vi "S4GUI.vi"(7 "Tab ObsEng":enum32{"Obs", "CCD modes", "Eng"}(tab)) -> ()   [LabVIEW 2018] (continued)
        n3639 = call-dynamic "Read Channel.vi"("error in (no error)"=w8486, "Acquisition in"=w8487) -> ("error out"=w8475:errorcluster, "Channel.lvclass"=w8476:refnum<class "Channel.lvclass">, "Acquisition out"=w8477:refnum<class "Acquisition.lvclass">)  [unwired: 7 in]
        n3640 = call-dynamic "Read Interface.vi"("error in (no error)"=w8475, "Channel in"=w8476) -> ("error out"=w8481:errorcluster, "Interface.lvclass"=w8482:refnum<class "Interface.lvclass">, "Channel out"=w8480:refnum<class "Channel.lvclass">)  [unwired: 7 in]
        n3641 = call "Write Exposure Time.vi"("error in (no error)"=w8481, "Exposure Time"=w8472, "Interface in"=w8482) -> ("error out"=w8473:errorcluster, "Interface out"=w8474:refnum<class "Interface.lvclass">)  [unwired: 7 in]
        n3642 = call-dynamic "Write Interface.vi"("error in (no error)"=w8473, "Interface.lvclass"=w8474, "Channel in"=w8480) -> ("error out"=w8479:errorcluster, "Channel out"=w8478:refnum<class "Channel.lvclass">)  [unwired: 7 in]
        n3643 = call-dynamic "Write Channel.vi"("error in (no error)"=w8479, "Channel.lvclass"=w8478, "Acquisition in"=w8477) -> ("error out"=w8483:errorcluster, "Acquisition out"=w8485:refnum<class "Acquisition.lvclass">)  [unwired: 7 in]
        n3644 = call-dynamic "Write AcquisitionD.vi"("error in (no error)"=w8483, "Acquisition.lvclass"=w8485, "S4ACS_GUI in"=w8484) -> ("error out"=w8469:errorcluster, "S4ACS_GUI out"=w8468:refnum<class "S4GUI.lvclass">)  [unwired: 7 in]
      }
      event "Stop ch1": Value Change {
        n3645 = event-data() -> ()  [unwired: 1 in, 6 out]
        n3646 = disable-structure shown="Enabled" {
          disable-tunnel: w8491 -> [w8524 w8552]
          disable-tunnel: w8490 -> [w8522 w8546]
          disable-tunnel: [w8504 w8545] -> w8489
          disable-tunnel: [w8492 w8552] -> w8488
          frame Disabled {
            # "Para movimento \nda lamina retardadora"
            # "Restaura a última sequência de lâminas"
            n3647 = call-dynamic "Read AcquisitionA.vi"("error in (no error)"=w8522, "S4ACS_GUI in"=w8524) -> ("error out"=w8526:errorcluster, "Acquisition.lvclass"=w8525:refnum<class "Acquisition.lvclass">, "S4ACS_GUI out"=w8523:refnum<class "S4GUI.lvclass">)  [unwired: 7 in]
            n3648 = disable-structure shown="Enabled" {
              disable-tunnel: w8526 -> [w8531 w8542]
              disable-tunnel: w8525 -> [w8530 w8543]
              disable-tunnel: [w8528 w8543] -> w8520
              disable-tunnel: [w8527 w8542] -> w8519
              frame Disabled {
                # "Só precisa enviar comando STOP quando\no controle dos ciclos for feito pelo ACS."
                n3649 = call-dynamic "Read Channel.vi"("error in (no error)"=w8531, "Acquisition in"=w8530) -> ("error out"=w8533:errorcluster, "Channel.lvclass"=w8532:refnum<class "Channel.lvclass">, "Acquisition out"=w8539:refnum<class "Acquisition.lvclass">)  [unwired: 7 in]
                n3650 = call-dynamic "Read State Machine.vi"("error in (no error)"=w8533, "Device in"=w8532) -> ("error out"=w8535:errorcluster, "State Machine.lvclass"=w8534:refnum<class "State Machine.lvclass">, "Device out"=w8537:refnum<class "Channel.lvclass">)  [unwired: 7 in]
                n3651 = call "Next State.vi"("error in (no error)"=w8535, "New_State"=u32 70, "State Machine in"=w8534) -> ("error out"=w8538:errorcluster, "State Machine out"=w8536:refnum<class "State Machine.lvclass">)  [unwired: 7 in]
                n3652 = call-dynamic "Write State Machine.vi"("error in (no error)"=w8538, "State Machine.lvclass"=w8536, "Device in"=w8537) -> ("error out"=w8540:errorcluster, "Device out"=w8541:refnum<class "Channel.lvclass">)  [unwired: 7 in]
                n3653 = call-dynamic "Write Channel.vi"("error in (no error)"=w8540, "Channel.lvclass"=w8541, "Acquisition in"=w8539) -> ("error out"=w8527:errorcluster, "Acquisition out"=w8528:refnum<class "Acquisition.lvclass">)  [unwired: 7 in]
              }
              frame Enabled {
                # "Não precisa enviar comando STOP para o ACS\nenquanto o controle dos ciclos for feito pela GUI."
              }
            }
            n3654 = call-dynamic "Write Acq_state.vi"("error in (no error)"=w8519, "Acq_state"=u32 0, "Acquisition in"=w8520) -> ("error out"=w8518:errorcluster, "Acquisition out"=w8517:refnum<class "Acquisition.lvclass">)  [unwired: 7 in]
            n3655 = call-dynamic "Write AcquisitionA.vi"("error in (no error)"=w8518, "Acquisition.lvclass"=w8517, "S4ACS_GUI in"=w8523) -> ("error out"=w8505:errorcluster, "S4ACS_GUI out"=w8503:refnum<class "S4GUI.lvclass">)  [unwired: 7 in]
            n3656 = call "Read Instrument.lvclass.vi"("error in (no error)"=w8505, "S4ACS_GUI in"=w8503) -> ("error out"=w8512:errorcluster, "Instrument.lvclass"=w8515:refnum<class "Instrument.lvclass">, "S4ACS_GUI out"=w8516:refnum<class "S4GUI.lvclass">)  [unwired: 7 in]
            n3657 = call "Read WPROT.vi"("error in (no error)"=w8512, "Instrument in"=w8515) -> ("error out"=w8511:errorcluster, "Opt_Selector.lvclass"=w8513:refnum<class "Opt_Selector.lvclass">, "Instrument out"=w8514:refnum<class "Instrument.lvclass">)  [unwired: 7 in]
            n3658 = call-dynamic "Read sequencia_ant.vi"("error in (no error)"=w8511, "Opt_Selector in"=w8513) -> ("error out"=w8507:errorcluster, "sequencia_ant"=w8506:u16, "Opt_Selector out"=w8508:refnum<class "Opt_Selector.lvclass">)  [unwired: 7 in]
            n3659 = call-dynamic "Write sequencia.vi"("error in (no error)"=w8507, "sequencia"=w8506, "Opt_Selector in"=w8508) -> ("error out"=w8494:errorcluster, "Opt_Selector out"=w8497:refnum<class "Opt_Selector.lvclass">)  [unwired: 7 in]
            n3660 = call-dynamic "Read State Machine.vi"("error in (no error)"=w8494, "Device in"=w8497) -> ("error out"=w8499:errorcluster, "State Machine.lvclass"=w8502:refnum<class "State Machine.lvclass">, "Device out"=w8496:refnum<class "Opt_Selector.lvclass">)  [unwired: 7 in]
            n3661 = call "Next State.vi"("error in (no error)"=w8499, "New_State"=10, "State Machine in"=w8502) -> ("error out"=w8498:errorcluster, "State Machine out"=w8501:refnum<class "State Machine.lvclass">)  [unwired: 7 in]
            n3662 = call-dynamic "Write State Machine.vi"("error in (no error)"=w8498, "State Machine.lvclass"=w8501, "Device in"=w8496) -> ("error out"=w8493:errorcluster, "Device out"=w8495:refnum<class "Opt_Selector.lvclass">)  [unwired: 7 in]
            n3663 = call "Write WPROT.vi"("error in (no error)"=w8493, "Opt_Selector.lvclass"=w8495, "Instrument in"=w8514) -> ("error out"=w8510:errorcluster, "Instrument out"=w8509:refnum<class "Instrument.lvclass">)  [unwired: 7 in]
            n3664 = call "Write Instrument.lvclass.vi"("error in (no error)"=w8510, "Instrument.lvclass"=w8509, "S4ACS_GUI in"=w8516) -> ("error out"=w8504:errorcluster, "S4ACS_GUI out"=w8492:refnum<class "S4GUI.lvclass">)  [unwired: 7 in]
          }
          frame Enabled {
            w8548 = FALSE ("Wait Until Done")
            n3665 = call <vilib>:"Application Directory.vi"() -> ("Application Directory"=w8544:path)
            n3666 = Build Path(base path=w8544, name or relative path="MsgStop1.vi") -> (appended path=w8551:path)
            n3667 = Open VI Reference(vi path=w8551, error in (no error)=w8546) -> (vi reference=w8550:refnum<vi>, error out=w8549:errorcluster)  [unwired: 4 in]
            n3668 = invoke class="VI" method="Run VI"(reference=w8550, error in=w8549, "Wait until done"=w8548, "Auto Dispose Ref"=w8548) -> (error out=w8545:errorcluster)  [unwired: 1 in, 4 out]
          }
        }
      }
      event "Stop ch2": Value Change {
        n3669 = event-data() -> ()  [unwired: 1 in, 6 out]
        n3670 = disable-structure shown="Enabled" {
          disable-tunnel: w8556 -> [w8589 w8610]
          disable-tunnel: w8555 -> [w8587 w8612]
          disable-tunnel: [w8569 w8611] -> w8554
          disable-tunnel: [w8557 w8610] -> w8553
          frame Disabled {
            # "Para movimento \nda lamina retardadora"
            # "Restaura a última sequência de lâminas"
            n3671 = call "Read AcquisitionB.vi"("error in (no error)"=w8587, "S4ACS_GUI in"=w8589) -> ("error out"=w8591:errorcluster, "Acquisition.lvclass"=w8590:refnum<class "Acquisition.lvclass">, "S4ACS_GUI out"=w8588:refnum<class "S4GUI.lvclass">)  [unwired: 7 in]
            n3672 = disable-structure shown="Enabled" {
              disable-tunnel: w8591 -> [w8596 w8607]
              disable-tunnel: w8590 -> [w8595 w8608]
              disable-tunnel: [w8593 w8608] -> w8585
              disable-tunnel: [w8592 w8607] -> w8584
              frame Disabled {
                # "Só precisa enviar comando STOP quando\no controle dos ciclos for feito pelo ACS."
                n3673 = call-dynamic "Read Channel.vi"("error in (no error)"=w8596, "Acquisition in"=w8595) -> ("error out"=w8598:errorcluster, "Channel.lvclass"=w8597:refnum<class "Channel.lvclass">, "Acquisition out"=w8604:refnum<class "Acquisition.lvclass">)  [unwired: 7 in]
                n3674 = call-dynamic "Read State Machine.vi"("error in (no error)"=w8598, "Device in"=w8597) -> ("error out"=w8600:errorcluster, "State Machine.lvclass"=w8599:refnum<class "State Machine.lvclass">, "Device out"=w8602:refnum<class "Channel.lvclass">)  [unwired: 7 in]
                n3675 = call "Next State.vi"("error in (no error)"=w8600, "New_State"=u32 70, "State Machine in"=w8599) -> ("error out"=w8603:errorcluster, "State Machine out"=w8601:refnum<class "State Machine.lvclass">)  [unwired: 7 in]
                n3676 = call-dynamic "Write State Machine.vi"("error in (no error)"=w8603, "State Machine.lvclass"=w8601, "Device in"=w8602) -> ("error out"=w8605:errorcluster, "Device out"=w8606:refnum<class "Channel.lvclass">)  [unwired: 7 in]
                n3677 = call-dynamic "Write Channel.vi"("error in (no error)"=w8605, "Channel.lvclass"=w8606, "Acquisition in"=w8604) -> ("error out"=w8592:errorcluster, "Acquisition out"=w8593:refnum<class "Acquisition.lvclass">)  [unwired: 7 in]
              }
              frame Enabled {
                # "Não precisa enviar comando STOP para o ACS\nenquanto o controle dos ciclos for feito pela GUI."
              }
            }
            n3678 = call-dynamic "Write Acq_state.vi"("error in (no error)"=w8584, "Acq_state"=u32 0, "Acquisition in"=w8585) -> ("error out"=w8583:errorcluster, "Acquisition out"=w8582:refnum<class "Acquisition.lvclass">)  [unwired: 7 in]
            n3679 = call "Write AcquisitionB.vi"("error in (no error)"=w8583, "Acquisition.lvclass"=w8582, "S4ACS_GUI in"=w8588) -> ("error out"=w8570:errorcluster, "S4ACS_GUI out"=w8568:refnum<class "S4GUI.lvclass">)  [unwired: 7 in]
            n3680 = call "Read Instrument.lvclass.vi"("error in (no error)"=w8570, "S4ACS_GUI in"=w8568) -> ("error out"=w8577:errorcluster, "Instrument.lvclass"=w8580:refnum<class "Instrument.lvclass">, "S4ACS_GUI out"=w8581:refnum<class "S4GUI.lvclass">)  [unwired: 7 in]
            n3681 = call "Read WPROT.vi"("error in (no error)"=w8577, "Instrument in"=w8580) -> ("error out"=w8576:errorcluster, "Opt_Selector.lvclass"=w8578:refnum<class "Opt_Selector.lvclass">, "Instrument out"=w8579:refnum<class "Instrument.lvclass">)  [unwired: 7 in]
            n3682 = call-dynamic "Read sequencia_ant.vi"("error in (no error)"=w8576, "Opt_Selector in"=w8578) -> ("error out"=w8572:errorcluster, "sequencia_ant"=w8571:u16, "Opt_Selector out"=w8573:refnum<class "Opt_Selector.lvclass">)  [unwired: 7 in]
            n3683 = call-dynamic "Write sequencia.vi"("error in (no error)"=w8572, "sequencia"=w8571, "Opt_Selector in"=w8573) -> ("error out"=w8559:errorcluster, "Opt_Selector out"=w8562:refnum<class "Opt_Selector.lvclass">)  [unwired: 7 in]
            n3684 = call-dynamic "Read State Machine.vi"("error in (no error)"=w8559, "Device in"=w8562) -> ("error out"=w8564:errorcluster, "State Machine.lvclass"=w8567:refnum<class "State Machine.lvclass">, "Device out"=w8561:refnum<class "Opt_Selector.lvclass">)  [unwired: 7 in]
            n3685 = call "Next State.vi"("error in (no error)"=w8564, "New_State"=10, "State Machine in"=w8567) -> ("error out"=w8563:errorcluster, "State Machine out"=w8566:refnum<class "State Machine.lvclass">)  [unwired: 7 in]
            n3686 = call-dynamic "Write State Machine.vi"("error in (no error)"=w8563, "State Machine.lvclass"=w8566, "Device in"=w8561) -> ("error out"=w8558:errorcluster, "Device out"=w8560:refnum<class "Opt_Selector.lvclass">)  [unwired: 7 in]
            n3687 = call "Write WPROT.vi"("error in (no error)"=w8558, "Opt_Selector.lvclass"=w8560, "Instrument in"=w8579) -> ("error out"=w8575:errorcluster, "Instrument out"=w8574:refnum<class "Instrument.lvclass">)  [unwired: 7 in]
            n3688 = call "Write Instrument.lvclass.vi"("error in (no error)"=w8575, "Instrument.lvclass"=w8574, "S4ACS_GUI in"=w8581) -> ("error out"=w8569:errorcluster, "S4ACS_GUI out"=w8557:refnum<class "S4GUI.lvclass">)  [unwired: 7 in]
          }
          frame Enabled {
            w8614 = FALSE ("Wait Until Done")
            n3689 = call <vilib>:"Application Directory.vi"() -> ("Application Directory"=w8609:path)
            n3690 = Build Path(base path=w8609, name or relative path="MsgStop2.vi") -> (appended path=w8617:path)
            n3691 = Open VI Reference(vi path=w8617, error in (no error)=w8612) -> (vi reference=w8616:refnum<vi>, error out=w8615:errorcluster)  [unwired: 4 in]
            n3692 = invoke class="VI" method="Run VI"(reference=w8616, error in=w8615, "Wait until done"=w8614, "Auto Dispose Ref"=w8614) -> (error out=w8611:errorcluster)  [unwired: 1 in, 4 out]
          }
        }
      }
      event "Stop ch3": Value Change {
        n3693 = event-data() -> ()  [unwired: 1 in, 6 out]
        n3694 = disable-structure shown="Enabled" {
          disable-tunnel: w8621 -> [w8654 w8675]
          disable-tunnel: w8620 -> [w8652 w8677]
          disable-tunnel: [w8634 w8676] -> w8619
          disable-tunnel: [w8622 w8675] -> w8618
          frame Disabled {
            # "Para movimento \nda lamina retardadora"
            # "Restaura a última sequência de lâminas"
            n3695 = call-dynamic "Read AcquisitionC.vi"("error in (no error)"=w8652, "S4ACS_GUI in"=w8654) -> ("error out"=w8656:errorcluster, "Acquisition.lvclass"=w8655:refnum<class "Acquisition.lvclass">, "S4ACS_GUI out"=w8653:refnum<class "S4GUI.lvclass">)  [unwired: 7 in]
            n3696 = disable-structure shown="Enabled" {
              disable-tunnel: w8656 -> [w8661 w8672]
              disable-tunnel: w8655 -> [w8660 w8673]
              disable-tunnel: [w8658 w8673] -> w8650
              disable-tunnel: [w8657 w8672] -> w8649
              frame Disabled {
                # "Só precisa enviar comando STOP quando\no controle dos ciclos for feito pelo ACS."
                n3697 = call-dynamic "Read Channel.vi"("error in (no error)"=w8661, "Acquisition in"=w8660) -> ("error out"=w8663:errorcluster, "Channel.lvclass"=w8662:refnum<class "Channel.lvclass">, "Acquisition out"=w8669:refnum<class "Acquisition.lvclass">)  [unwired: 7 in]
                n3698 = call-dynamic "Read State Machine.vi"("error in (no error)"=w8663, "Device in"=w8662) -> ("error out"=w8665:errorcluster, "State Machine.lvclass"=w8664:refnum<class "State Machine.lvclass">, "Device out"=w8667:refnum<class "Channel.lvclass">)  [unwired: 7 in]
                n3699 = call "Next State.vi"("error in (no error)"=w8665, "New_State"=u32 70, "State Machine in"=w8664) -> ("error out"=w8668:errorcluster, "State Machine out"=w8666:refnum<class "State Machine.lvclass">)  [unwired: 7 in]
                n3700 = call-dynamic "Write State Machine.vi"("error in (no error)"=w8668, "State Machine.lvclass"=w8666, "Device in"=w8667) -> ("error out"=w8670:errorcluster, "Device out"=w8671:refnum<class "Channel.lvclass">)  [unwired: 7 in]
                n3701 = call-dynamic "Write Channel.vi"("error in (no error)"=w8670, "Channel.lvclass"=w8671, "Acquisition in"=w8669) -> ("error out"=w8657:errorcluster, "Acquisition out"=w8658:refnum<class "Acquisition.lvclass">)  [unwired: 7 in]
              }
              frame Enabled {
                # "Não precisa enviar comando STOP para o ACS\nenquanto o controle dos ciclos for feito pela GUI."
              }
            }
            n3702 = call-dynamic "Write Acq_state.vi"("error in (no error)"=w8649, "Acq_state"=u32 0, "Acquisition in"=w8650) -> ("error out"=w8648:errorcluster, "Acquisition out"=w8647:refnum<class "Acquisition.lvclass">)  [unwired: 7 in]
            n3703 = call-dynamic "Write AcquisitionC.vi"("error in (no error)"=w8648, "Acquisition.lvclass"=w8647, "S4ACS_GUI in"=w8653) -> ("error out"=w8635:errorcluster, "S4ACS_GUI out"=w8633:refnum<class "S4GUI.lvclass">)  [unwired: 7 in]
            n3704 = call "Read Instrument.lvclass.vi"("error in (no error)"=w8635, "S4ACS_GUI in"=w8633) -> ("error out"=w8642:errorcluster, "Instrument.lvclass"=w8645:refnum<class "Instrument.lvclass">, "S4ACS_GUI out"=w8646:refnum<class "S4GUI.lvclass">)  [unwired: 7 in]
            n3705 = call "Read WPROT.vi"("error in (no error)"=w8642, "Instrument in"=w8645) -> ("error out"=w8641:errorcluster, "Opt_Selector.lvclass"=w8643:refnum<class "Opt_Selector.lvclass">, "Instrument out"=w8644:refnum<class "Instrument.lvclass">)  [unwired: 7 in]
            n3706 = call-dynamic "Read sequencia_ant.vi"("error in (no error)"=w8641, "Opt_Selector in"=w8643) -> ("error out"=w8637:errorcluster, "sequencia_ant"=w8636:u16, "Opt_Selector out"=w8638:refnum<class "Opt_Selector.lvclass">)  [unwired: 7 in]
            n3707 = call-dynamic "Write sequencia.vi"("error in (no error)"=w8637, "sequencia"=w8636, "Opt_Selector in"=w8638) -> ("error out"=w8624:errorcluster, "Opt_Selector out"=w8627:refnum<class "Opt_Selector.lvclass">)  [unwired: 7 in]
            n3708 = call-dynamic "Read State Machine.vi"("error in (no error)"=w8624, "Device in"=w8627) -> ("error out"=w8629:errorcluster, "State Machine.lvclass"=w8632:refnum<class "State Machine.lvclass">, "Device out"=w8626:refnum<class "Opt_Selector.lvclass">)  [unwired: 7 in]
            n3709 = call "Next State.vi"("error in (no error)"=w8629, "New_State"=10, "State Machine in"=w8632) -> ("error out"=w8628:errorcluster, "State Machine out"=w8631:refnum<class "State Machine.lvclass">)  [unwired: 7 in]
            n3710 = call-dynamic "Write State Machine.vi"("error in (no error)"=w8628, "State Machine.lvclass"=w8631, "Device in"=w8626) -> ("error out"=w8623:errorcluster, "Device out"=w8625:refnum<class "Opt_Selector.lvclass">)  [unwired: 7 in]
            n3711 = call "Write WPROT.vi"("error in (no error)"=w8623, "Opt_Selector.lvclass"=w8625, "Instrument in"=w8644) -> ("error out"=w8640:errorcluster, "Instrument out"=w8639:refnum<class "Instrument.lvclass">)  [unwired: 7 in]
            n3712 = call "Write Instrument.lvclass.vi"("error in (no error)"=w8640, "Instrument.lvclass"=w8639, "S4ACS_GUI in"=w8646) -> ("error out"=w8634:errorcluster, "S4ACS_GUI out"=w8622:refnum<class "S4GUI.lvclass">)  [unwired: 7 in]
          }
          frame Enabled {
            w8679 = FALSE ("Wait Until Done")
            n3713 = call <vilib>:"Application Directory.vi"() -> ("Application Directory"=w8674:path)
            n3714 = Build Path(base path=w8674, name or relative path="MsgStop3.vi") -> (appended path=w8682:path)
            n3715 = Open VI Reference(vi path=w8682, error in (no error)=w8677) -> (vi reference=w8681:refnum<vi>, error out=w8680:errorcluster)  [unwired: 4 in]
            n3716 = invoke class="VI" method="Run VI"(reference=w8681, error in=w8680, "Wait until done"=w8679, "Auto Dispose Ref"=w8679) -> (error out=w8676:errorcluster)  [unwired: 1 in, 4 out]
          }
        }
      }
      event "Stop ch4": Value Change {
        n3717 = event-data() -> ()  [unwired: 1 in, 6 out]
        n3718 = disable-structure shown="Enabled" {
          disable-tunnel: w8686 -> [w8719 w8740]
          disable-tunnel: w8685 -> [w8717 w8742]
          disable-tunnel: [w8699 w8741] -> w8684
          disable-tunnel: [w8687 w8740] -> w8683
          frame Disabled {
            # "Para movimento \nda lamina retardadora"
            # "Restaura a última sequência de lâminas"
            n3719 = call-dynamic "Read AcquisitionD.vi"("error in (no error)"=w8717, "S4ACS_GUI in"=w8719) -> ("error out"=w8721:errorcluster, "Acquisition.lvclass"=w8720:refnum<class "Acquisition.lvclass">, "S4ACS_GUI out"=w8718:refnum<class "S4GUI.lvclass">)  [unwired: 7 in]
            n3720 = disable-structure shown="Enabled" {
              disable-tunnel: w8721 -> [w8726 w8737]
              disable-tunnel: w8720 -> [w8725 w8738]
              disable-tunnel: [w8723 w8738] -> w8715
              disable-tunnel: [w8722 w8737] -> w8714
              frame Disabled {
                # "Só precisa enviar comando STOP quando\no controle dos ciclos for feito pelo ACS."
                n3721 = call-dynamic "Read Channel.vi"("error in (no error)"=w8726, "Acquisition in"=w8725) -> ("error out"=w8728:errorcluster, "Channel.lvclass"=w8727:refnum<class "Channel.lvclass">, "Acquisition out"=w8734:refnum<class "Acquisition.lvclass">)  [unwired: 7 in]
                n3722 = call-dynamic "Read State Machine.vi"("error in (no error)"=w8728, "Device in"=w8727) -> ("error out"=w8730:errorcluster, "State Machine.lvclass"=w8729:refnum<class "State Machine.lvclass">, "Device out"=w8732:refnum<class "Channel.lvclass">)  [unwired: 7 in]
                n3723 = call "Next State.vi"("error in (no error)"=w8730, "New_State"=u32 70, "State Machine in"=w8729) -> ("error out"=w8733:errorcluster, "State Machine out"=w8731:refnum<class "State Machine.lvclass">)  [unwired: 7 in]
                n3724 = call-dynamic "Write State Machine.vi"("error in (no error)"=w8733, "State Machine.lvclass"=w8731, "Device in"=w8732) -> ("error out"=w8735:errorcluster, "Device out"=w8736:refnum<class "Channel.lvclass">)  [unwired: 7 in]
                n3725 = call-dynamic "Write Channel.vi"("error in (no error)"=w8735, "Channel.lvclass"=w8736, "Acquisition in"=w8734) -> ("error out"=w8722:errorcluster, "Acquisition out"=w8723:refnum<class "Acquisition.lvclass">)  [unwired: 7 in]
              }
              frame Enabled {
                # "Não precisa enviar comando STOP para o ACS\nenquanto o controle dos ciclos for feito pela GUI."
              }
            }
            n3726 = call-dynamic "Write Acq_state.vi"("error in (no error)"=w8714, "Acq_state"=u32 0, "Acquisition in"=w8715) -> ("error out"=w8713:errorcluster, "Acquisition out"=w8712:refnum<class "Acquisition.lvclass">)  [unwired: 7 in]
            n3727 = call-dynamic "Write AcquisitionD.vi"("error in (no error)"=w8713, "Acquisition.lvclass"=w8712, "S4ACS_GUI in"=w8718) -> ("error out"=w8700:errorcluster, "S4ACS_GUI out"=w8698:refnum<class "S4GUI.lvclass">)  [unwired: 7 in]
            n3728 = call "Read Instrument.lvclass.vi"("error in (no error)"=w8700, "S4ACS_GUI in"=w8698) -> ("error out"=w8707:errorcluster, "Instrument.lvclass"=w8710:refnum<class "Instrument.lvclass">, "S4ACS_GUI out"=w8711:refnum<class "S4GUI.lvclass">)  [unwired: 7 in]
            n3729 = call "Read WPROT.vi"("error in (no error)"=w8707, "Instrument in"=w8710) -> ("error out"=w8706:errorcluster, "Opt_Selector.lvclass"=w8708:refnum<class "Opt_Selector.lvclass">, "Instrument out"=w8709:refnum<class "Instrument.lvclass">)  [unwired: 7 in]
            n3730 = call-dynamic "Read sequencia_ant.vi"("error in (no error)"=w8706, "Opt_Selector in"=w8708) -> ("error out"=w8702:errorcluster, "sequencia_ant"=w8701:u16, "Opt_Selector out"=w8703:refnum<class "Opt_Selector.lvclass">)  [unwired: 7 in]
            n3731 = call-dynamic "Write sequencia.vi"("error in (no error)"=w8702, "sequencia"=w8701, "Opt_Selector in"=w8703) -> ("error out"=w8689:errorcluster, "Opt_Selector out"=w8692:refnum<class "Opt_Selector.lvclass">)  [unwired: 7 in]
            n3732 = call-dynamic "Read State Machine.vi"("error in (no error)"=w8689, "Device in"=w8692) -> ("error out"=w8694:errorcluster, "State Machine.lvclass"=w8697:refnum<class "State Machine.lvclass">, "Device out"=w8691:refnum<class "Opt_Selector.lvclass">)  [unwired: 7 in]
            n3733 = call "Next State.vi"("error in (no error)"=w8694, "New_State"=10, "State Machine in"=w8697) -> ("error out"=w8693:errorcluster, "State Machine out"=w8696:refnum<class "State Machine.lvclass">)  [unwired: 7 in]
            n3734 = call-dynamic "Write State Machine.vi"("error in (no error)"=w8693, "State Machine.lvclass"=w8696, "Device in"=w8691) -> ("error out"=w8688:errorcluster, "Device out"=w8690:refnum<class "Opt_Selector.lvclass">)  [unwired: 7 in]
            n3735 = call "Write WPROT.vi"("error in (no error)"=w8688, "Opt_Selector.lvclass"=w8690, "Instrument in"=w8709) -> ("error out"=w8705:errorcluster, "Instrument out"=w8704:refnum<class "Instrument.lvclass">)  [unwired: 7 in]
            n3736 = call "Write Instrument.lvclass.vi"("error in (no error)"=w8705, "Instrument.lvclass"=w8704, "S4ACS_GUI in"=w8711) -> ("error out"=w8699:errorcluster, "S4ACS_GUI out"=w8687:refnum<class "S4GUI.lvclass">)  [unwired: 7 in]
          }
          frame Enabled {
            w8744 = FALSE ("Wait Until Done")
            n3737 = call <vilib>:"Application Directory.vi"() -> ("Application Directory"=w8739:path)
            n3738 = Build Path(base path=w8739, name or relative path="MsgStop4.vi") -> (appended path=w8747:path)
            n3739 = Open VI Reference(vi path=w8747, error in (no error)=w8742) -> (vi reference=w8746:refnum<vi>, error out=w8745:errorcluster)  [unwired: 4 in]
            n3740 = invoke class="VI" method="Run VI"(reference=w8746, error in=w8745, "Wait until done"=w8744, "Auto Dispose Ref"=w8744) -> (error out=w8741:errorcluster)  [unwired: 1 in, 4 out]
          }
        }
      }
      event "Pause ch1": Value Change {
        n3741 = event-data() -> ()  [unwired: 1 in, 6 out]
        n3742 = disable-structure shown="Enabled" {
          disable-tunnel: w8751 -> [w8767 w8779]
          disable-tunnel: [w8765 w8777] -> w8750
          disable-tunnel: w8749 -> [w8764 w8778]
          disable-tunnel: [w8752 w8779] -> w8748
          frame Disabled {
            n3743 = call-dynamic "Read AcquisitionA.vi"("error in (no error)"=w8764, "S4ACS_GUI in"=w8767) -> ("error out"=w8759:errorcluster, "Acquisition.lvclass"=w8758:refnum<class "Acquisition.lvclass">, "S4ACS_GUI out"=w8766:refnum<class "S4GUI.lvclass">)  [unwired: 7 in]
            n3744 = call-dynamic "Read Acq_state.vi"("error in (no error)"=w8759, "Acquisition in"=w8758) -> ("error out"=w8761:errorcluster, "Acq_state"=w8762:u32, "Acquisition out"=w8763:refnum<class "Acquisition.lvclass">)  [unwired: 7 in]
            n3745 = call-dynamic "Write Acq_prevstate.vi"("error in (no error)"=w8761, "Acq_prevstate"=w8762, "Acquisition in"=w8763) -> ("error out"=w8756:errorcluster, "Acquisition out"=w8757:refnum<class "Acquisition.lvclass">)  [unwired: 7 in]
            n3746 = call-dynamic "Write Acq_state.vi"("error in (no error)"=w8756, "Acq_state"=u32 400, "Acquisition in"=w8757) -> ("error out"=w8754:errorcluster, "Acquisition out"=w8755:refnum<class "Acquisition.lvclass">)  [unwired: 7 in]
            n3747 = disable-structure shown="Enabled" {
              disable-tunnel: w8754 -> [w8769 w8775]
              disable-tunnel: [w8768 w8775] -> w8753
              frame Disabled {
                n3748 = property on="Start ch1" class="Bool"(error in=w8769, "BoolText.Text"="RESUME" ("Caption.Text")) -> (error out=w8773:errorcluster)  [unwired: 1 in, 1 out]
                n3749 = property on="Pause ch1" class="Bool"(error in=w8773, "DisabledEnum"=T12."Disabled and Grayed Out" ("Disabled")) -> (error out=w8774:errorcluster)  [unwired: 1 in, 1 out]
                n3750 = property on="Start ch1" class="Bool"(error in=w8774, "DisabledEnum"=T12."Enabled" ("Disabled")) -> (error out=w8768:errorcluster)  [unwired: 1 in, 1 out]
              }
              frame Enabled {
              }
            }
            n3751 = call-dynamic "Write AcquisitionA.vi"("error in (no error)"=w8753, "Acquisition.lvclass"=w8755, "S4ACS_GUI in"=w8766) -> ("error out"=w8765:errorcluster, "S4ACS_GUI out"=w8752:refnum<class "S4GUI.lvclass">)  [unwired: 7 in]
          }
          frame Enabled {
            w8781 = FALSE ("Wait Until Done")
            n3752 = call <vilib>:"Application Directory.vi"() -> ("Application Directory"=w8776:path)
            n3753 = Build Path(base path=w8776, name or relative path="MsgPause1.vi") -> (appended path=w8784:path)
            n3754 = Open VI Reference(vi path=w8784, error in (no error)=w8778) -> (vi reference=w8783:refnum<vi>, error out=w8782:errorcluster)  [unwired: 4 in]
            n3755 = invoke class="VI" method="Run VI"(reference=w8783, error in=w8782, "Wait until done"=w8781, "Auto Dispose Ref"=w8781) -> (error out=w8777:errorcluster)  [unwired: 1 in, 4 out]
          }
        }
      }
      event "Pause ch2": Value Change {
        n3756 = event-data() -> ()  [unwired: 1 in, 6 out]
        n3757 = disable-structure shown="Enabled" {
          disable-tunnel: w8788 -> [w8803 w8805]
          disable-tunnel: [w8801 w8806] -> w8787
          disable-tunnel: w8786 -> [w8800 w8807]
          disable-tunnel: [w8790 w8805] -> w8785
          frame Disabled {
            n3758 = call "Read AcquisitionB.vi"("error in (no error)"=w8800, "S4ACS_GUI in"=w8803) -> ("error out"=w8795:errorcluster, "Acquisition.lvclass"=w8794:refnum<class "Acquisition.lvclass">, "S4ACS_GUI out"=w8802:refnum<class "S4GUI.lvclass">)  [unwired: 7 in]
            n3759 = call-dynamic "Read Acq_state.vi"("error in (no error)"=w8795, "Acquisition in"=w8794) -> ("error out"=w8797:errorcluster, "Acq_state"=w8798:u32, "Acquisition out"=w8799:refnum<class "Acquisition.lvclass">)  [unwired: 7 in]
            n3760 = call-dynamic "Write Acq_prevstate.vi"("error in (no error)"=w8797, "Acq_prevstate"=w8798, "Acquisition in"=w8799) -> ("error out"=w8792:errorcluster, "Acquisition out"=w8793:refnum<class "Acquisition.lvclass">)  [unwired: 7 in]
            n3761 = call-dynamic "Write Acq_state.vi"("error in (no error)"=w8792, "Acq_state"=u32 400, "Acquisition in"=w8793) -> ("error out"=w8789:errorcluster, "Acquisition out"=w8791:refnum<class "Acquisition.lvclass">)  [unwired: 7 in]
            n3762 = call "Write AcquisitionB.vi"("error in (no error)"=w8789, "Acquisition.lvclass"=w8791, "S4ACS_GUI in"=w8802) -> ("error out"=w8801:errorcluster, "S4ACS_GUI out"=w8790:refnum<class "S4GUI.lvclass">)  [unwired: 7 in]
          }
          frame Enabled {
            w8809 = FALSE ("Wait Until Done")
            n3763 = call <vilib>:"Application Directory.vi"() -> ("Application Directory"=w8804:path)
            n3764 = Build Path(base path=w8804, name or relative path="MsgPause2.vi") -> (appended path=w8812:path)
            n3765 = Open VI Reference(vi path=w8812, error in (no error)=w8807) -> (vi reference=w8811:refnum<vi>, error out=w8810:errorcluster)  [unwired: 4 in]
            n3766 = invoke class="VI" method="Run VI"(reference=w8811, error in=w8810, "Wait until done"=w8809, "Auto Dispose Ref"=w8809) -> (error out=w8806:errorcluster)  [unwired: 1 in, 4 out]
          }
        }
      }
      event "Pause ch3": Value Change {
        n3767 = event-data() -> ()  [unwired: 1 in, 6 out]
        n3768 = disable-structure shown="Enabled" {
          disable-tunnel: w8816 -> [w8831 w8833]
          disable-tunnel: [w8829 w8834] -> w8815
          disable-tunnel: w8814 -> [w8828 w8835]
          disable-tunnel: [w8818 w8833] -> w8813
          frame Disabled {
            n3769 = call-dynamic "Read AcquisitionC.vi"("error in (no error)"=w8828, "S4ACS_GUI in"=w8831) -> ("error out"=w8823:errorcluster, "Acquisition.lvclass"=w8822:refnum<class "Acquisition.lvclass">, "S4ACS_GUI out"=w8830:refnum<class "S4GUI.lvclass">)  [unwired: 7 in]
            n3770 = call-dynamic "Read Acq_state.vi"("error in (no error)"=w8823, "Acquisition in"=w8822) -> ("error out"=w8825:errorcluster, "Acq_state"=w8826:u32, "Acquisition out"=w8827:refnum<class "Acquisition.lvclass">)  [unwired: 7 in]
            n3771 = call-dynamic "Write Acq_prevstate.vi"("error in (no error)"=w8825, "Acq_prevstate"=w8826, "Acquisition in"=w8827) -> ("error out"=w8820:errorcluster, "Acquisition out"=w8821:refnum<class "Acquisition.lvclass">)  [unwired: 7 in]
            n3772 = call-dynamic "Write Acq_state.vi"("error in (no error)"=w8820, "Acq_state"=u32 400, "Acquisition in"=w8821) -> ("error out"=w8817:errorcluster, "Acquisition out"=w8819:refnum<class "Acquisition.lvclass">)  [unwired: 7 in]
            n3773 = call-dynamic "Write AcquisitionC.vi"("error in (no error)"=w8817, "Acquisition.lvclass"=w8819, "S4ACS_GUI in"=w8830) -> ("error out"=w8829:errorcluster, "S4ACS_GUI out"=w8818:refnum<class "S4GUI.lvclass">)  [unwired: 7 in]
          }
          frame Enabled {
            w8837 = FALSE ("Wait Until Done")
            n3774 = call <vilib>:"Application Directory.vi"() -> ("Application Directory"=w8832:path)
            n3775 = Build Path(base path=w8832, name or relative path="MsgPause3.vi") -> (appended path=w8840:path)
            n3776 = Open VI Reference(vi path=w8840, error in (no error)=w8835) -> (vi reference=w8839:refnum<vi>, error out=w8838:errorcluster)  [unwired: 4 in]
            n3777 = invoke class="VI" method="Run VI"(reference=w8839, error in=w8838, "Wait until done"=w8837, "Auto Dispose Ref"=w8837) -> (error out=w8834:errorcluster)  [unwired: 1 in, 4 out]
          }
        }
      }
      event "Pause ch4": Value Change {
        n3778 = event-data() -> ()  [unwired: 1 in, 6 out]
        n3779 = disable-structure shown="Enabled" {
          disable-tunnel: w8844 -> [w8859 w8868]
          disable-tunnel: [w8857 w8861] -> w8843
          disable-tunnel: w8842 -> [w8856 w8862]
          disable-tunnel: [w8846 w8868] -> w8841
          frame Disabled {
            n3780 = call-dynamic "Read AcquisitionD.vi"("error in (no error)"=w8856, "S4ACS_GUI in"=w8859) -> ("error out"=w8851:errorcluster, "Acquisition.lvclass"=w8850:refnum<class "Acquisition.lvclass">, "S4ACS_GUI out"=w8858:refnum<class "S4GUI.lvclass">)  [unwired: 7 in]
            n3781 = call-dynamic "Read Acq_state.vi"("error in (no error)"=w8851, "Acquisition in"=w8850) -> ("error out"=w8853:errorcluster, "Acq_state"=w8854:u32, "Acquisition out"=w8855:refnum<class "Acquisition.lvclass">)  [unwired: 7 in]
            n3782 = call-dynamic "Write Acq_prevstate.vi"("error in (no error)"=w8853, "Acq_prevstate"=w8854, "Acquisition in"=w8855) -> ("error out"=w8848:errorcluster, "Acquisition out"=w8849:refnum<class "Acquisition.lvclass">)  [unwired: 7 in]
            n3783 = call-dynamic "Write Acq_state.vi"("error in (no error)"=w8848, "Acq_state"=u32 400, "Acquisition in"=w8849) -> ("error out"=w8845:errorcluster, "Acquisition out"=w8847:refnum<class "Acquisition.lvclass">)  [unwired: 7 in]
            n3784 = call-dynamic "Write AcquisitionD.vi"("error in (no error)"=w8845, "Acquisition.lvclass"=w8847, "S4ACS_GUI in"=w8858) -> ("error out"=w8857:errorcluster, "S4ACS_GUI out"=w8846:refnum<class "S4GUI.lvclass">)  [unwired: 7 in]
          }
          frame Enabled {
            w8864 = FALSE ("Wait Until Done")
            n3785 = call <vilib>:"Application Directory.vi"() -> ("Application Directory"=w8860:path)
            n3786 = Build Path(base path=w8860, name or relative path="MsgPause4.vi") -> (appended path=w8867:path)
            n3787 = Open VI Reference(vi path=w8867, error in (no error)=w8862) -> (vi reference=w8866:refnum<vi>, error out=w8865:errorcluster)  [unwired: 4 in]
            n3788 = invoke class="VI" method="Run VI"(reference=w8866, error in=w8865, "Wait until done"=w8864, "Auto Dispose Ref"=w8864) -> (error out=w8861:errorcluster)  [unwired: 1 in, 4 out]
          }
        }
      }
      event "Stop SM": Value Change {
        w8874 = 0.0 ("Scale.Range:Minor Increment")
        n3789 = event-data() -> ()  [unwired: 1 in, 6 out]
        n3790 = call-dynamic "Write User Event.vi"("error in (no error)"=w8872, "User Event"="STOP SM CLICKED", "S4GUI in"=w8873) -> ("error out"=w8870:errorcluster, "S4GUI out"=w8871:refnum<class "S4GUI.lvclass">)  [unwired: 7 in]
        n3791 = disable-structure shown="Enabled" {
          disable-tunnel: w8871 -> [w8911 w8935]
          disable-tunnel: w8870 -> [w8909 w8936]
          disable-tunnel: [w8896 w8934] -> w8876
          disable-tunnel: [w8880 w8935] -> w8875
          frame Disabled {
            # "Não precisa enviar comando STOP para o ACS\nenquanto o controle dos ciclos for feito pela GUI."
            # "Para movimento \nda lamina retardadora"
            # "Restaura a sequencia anterior"
            n3792 = call-dynamic "Read AcquisitionA.vi"("error in (no error)"=w8909, "S4ACS_GUI in"=w8911) -> ("error out"=w8913:errorcluster, "Acquisition.lvclass"=w8912:refnum<class "Acquisition.lvclass">, "S4ACS_GUI out"=w8910:refnum<class "S4GUI.lvclass">)  [unwired: 7 in]
            n3793 = disable-structure shown="Enabled" {
              disable-tunnel: [w8927 w8931] -> w8915
              disable-tunnel: [w8926 w8932] -> w8914
              disable-tunnel: w8913 -> [w8918 w8931]
              disable-tunnel: w8912 -> [w8917 w8932]
              frame Disabled {
                n3794 = call-dynamic "Read Channel.vi"("error in (no error)"=w8918, "Acquisition in"=w8917) -> ("error out"=w8920:errorcluster, "Channel.lvclass"=w8919:refnum<class "Channel.lvclass">, "Acquisition out"=w8928:refnum<class "Acquisition.lvclass">)  [unwired: 7 in]
                n3795 = call-dynamic "Read State Machine.vi"("error in (no error)"=w8920, "Device in"=w8919) -> ("error out"=w8922:errorcluster, "State Machine.lvclass"=w8921:refnum<class "State Machine.lvclass">, "Device out"=w8924:refnum<class "Channel.lvclass">)  [unwired: 7 in]
                n3796 = call "Next State.vi"("error in (no error)"=w8922, "New_State"=u32 70, "State Machine in"=w8921) -> ("error out"=w8925:errorcluster, "State Machine out"=w8923:refnum<class "State Machine.lvclass">)  [unwired: 7 in]
                n3797 = call-dynamic "Write State Machine.vi"("error in (no error)"=w8925, "State Machine.lvclass"=w8923, "Device in"=w8924) -> ("error out"=w8929:errorcluster, "Device out"=w8930:refnum<class "Channel.lvclass">)  [unwired: 7 in]
                n3798 = call-dynamic "Write Channel.vi"("error in (no error)"=w8929, "Channel.lvclass"=w8930, "Acquisition in"=w8928) -> ("error out"=w8927:errorcluster, "Acquisition out"=w8926:refnum<class "Acquisition.lvclass">)  [unwired: 7 in]
              }
              frame Enabled {
              }
            }
            n3799 = call-dynamic "Write AcquisitionA.vi"("error in (no error)"=w8915, "Acquisition.lvclass"=w8914, "S4ACS_GUI in"=w8910) -> ("error out"=w8878:errorcluster, "S4ACS_GUI out"=w8879:refnum<class "S4GUI.lvclass">)  [unwired: 7 in]
            n3800 = call-dynamic "Write Obs_state.vi"("error in (no error)"=w8878, "Obs_state"=u32 0, "S4ACS_GUI in"=w8879) -> ("error out"=w8898:errorcluster, "S4ACS_GUI out"=w8899:refnum<class "S4GUI.lvclass">)  [unwired: 7 in]
            n3801 = call "Read Instrument.lvclass.vi"("error in (no error)"=w8898, "S4ACS_GUI in"=w8899) -> ("error out"=w8907:errorcluster, "Instrument.lvclass"=w8905:refnum<class "Instrument.lvclass">, "S4ACS_GUI out"=w8906:refnum<class "S4GUI.lvclass">)  [unwired: 7 in]
            n3802 = call "Read WPROT.vi"("error in (no error)"=w8907, "Instrument in"=w8905) -> ("error out"=w8892:errorcluster, "Opt_Selector.lvclass"=w8895:refnum<class "Opt_Selector.lvclass">, "Instrument out"=w8904:refnum<class "Instrument.lvclass">)  [unwired: 7 in]
            n3803 = call-dynamic "Read sequencia_ant.vi"("error in (no error)"=w8892, "Opt_Selector in"=w8895) -> ("error out"=w8891:errorcluster, "sequencia_ant"=w8893:u16, "Opt_Selector out"=w8894:refnum<class "Opt_Selector.lvclass">)  [unwired: 7 in]
            n3804 = call-dynamic "Write sequencia.vi"("error in (no error)"=w8891, "sequencia"=w8893, "Opt_Selector in"=w8894) -> ("error out"=w8889:errorcluster, "Opt_Selector out"=w8890:refnum<class "Opt_Selector.lvclass">)  [unwired: 7 in]
            n3805 = call-dynamic "Read State Machine.vi"("error in (no error)"=w8889, "Device in"=w8890) -> ("error out"=w8884:errorcluster, "State Machine.lvclass"=w8887:refnum<class "State Machine.lvclass">, "Device out"=w8888:refnum<class "Opt_Selector.lvclass">)  [unwired: 7 in]
            n3806 = call "Next State.vi"("error in (no error)"=w8884, "New_State"=10, "State Machine in"=w8887) -> ("error out"=w8883:errorcluster, "State Machine out"=w8886:refnum<class "State Machine.lvclass">)  [unwired: 7 in]
            n3807 = call-dynamic "Write State Machine.vi"("error in (no error)"=w8883, "State Machine.lvclass"=w8886, "Device in"=w8888) -> ("error out"=w8882:errorcluster, "Device out"=w8881:refnum<class "Opt_Selector.lvclass">)  [unwired: 7 in]
            n3808 = call "Write WPROT.vi"("error in (no error)"=w8882, "Opt_Selector.lvclass"=w8881, "Instrument in"=w8904) -> ("error out"=w8902:errorcluster, "Instrument out"=w8903:refnum<class "Instrument.lvclass">)  [unwired: 7 in]
            n3809 = call "Write Instrument.lvclass.vi"("error in (no error)"=w8902, "Instrument.lvclass"=w8903, "S4ACS_GUI in"=w8906) -> ("error out"=w8901:errorcluster, "S4ACS_GUI out"=w8900:refnum<class "S4GUI.lvclass">)  [unwired: 7 in]
            n3810 = call-dynamic "Write ciclos.vi"("error in (no error)"=w8901, "ciclos"=u32 0, "S4ACS_GUI in"=w8900) -> ("error out"=w8896:errorcluster, "S4ACS_GUI out"=w8880:refnum<class "S4GUI.lvclass">)  [unwired: 7 in]
          }
          frame Enabled {
            w8938 = FALSE ("Wait Until Done")
            n3811 = call <vilib>:"Application Directory.vi"() -> ("Application Directory"=w8933:path)
            n3812 = Build Path(base path=w8933, name or relative path="MsgStopSync.vi") -> (appended path=w8941:path)
            n3813 = Open VI Reference(vi path=w8941, error in (no error)=w8936) -> (vi reference=w8940:refnum<vi>, error out=w8939:errorcluster)  [unwired: 4 in]
            n3814 = invoke class="VI" method="Run VI"(reference=w8940, error in=w8939, "Wait until done"=w8938, "Auto Dispose Ref"=w8938) -> (error out=w8934:errorcluster)  [unwired: 1 in, 4 out]
          }
        }
        n3815 = property on="#Cycles Done" class="Slide (strict)"(error in=w8876, "Scale.Maximum"=w8874, "Scale.Minimum"=w8874) -> (error out=w8877:errorcluster)  [unwired: 1 in, 1 out]
      }
      event "Abort SM": Value Change {
        w8949 = 0.0 ("Scale.Range:Minor Increment")
        n3816 = event-data() -> ()  [unwired: 1 in, 6 out]
        n3817 = call-dynamic "Write User Event.vi"("error in (no error)"=w8945, "User Event"="ABORT SM CLICKED", "S4GUI in"=w8946) -> ("error out"=w8943:errorcluster, "S4GUI out"=w8944:refnum<class "S4GUI.lvclass">)  [unwired: 7 in]
        n3818 = disable-structure shown="Enabled" {
          disable-tunnel: w8944 -> [w9040 w9064]
          disable-tunnel: w8943 -> [w9038 w9066]
          disable-tunnel: [w8952 w9064] -> w8948
          disable-tunnel: [w8951 w9065] -> w8947
          frame Disabled {
            # "Restaura a sequencia anterior"
            # "Para movimento \nda lamina retardadora"
            n3819 = call-dynamic "Read AcquisitionA.vi"("error in (no error)"=w9038, "S4ACS_GUI in"=w9040) -> ("error out"=w9043:errorcluster, "Acquisition.lvclass"=w9042:refnum<class "Acquisition.lvclass">, "S4ACS_GUI out"=w9039:refnum<class "S4GUI.lvclass">)  [unwired: 7 in]
            n3820 = call-dynamic "Read Channel.vi"("error in (no error)"=w9043, "Acquisition in"=w9042) -> ("error out"=w9045:errorcluster, "Channel.lvclass"=w9044:refnum<class "Channel.lvclass">, "Acquisition out"=w9053:refnum<class "Acquisition.lvclass">)  [unwired: 7 in]
            n3821 = call-dynamic "Read State Machine.vi"("error in (no error)"=w9045, "Device in"=w9044) -> ("error out"=w9047:errorcluster, "State Machine.lvclass"=w9046:refnum<class "State Machine.lvclass">, "Device out"=w9049:refnum<class "Channel.lvclass">)  [unwired: 7 in]
            n3822 = call "Next State.vi"("error in (no error)"=w9047, "New_State"=u32 80, "State Machine in"=w9046) -> ("error out"=w9050:errorcluster, "State Machine out"=w9048:refnum<class "State Machine.lvclass">)  [unwired: 7 in]
            n3823 = call-dynamic "Write State Machine.vi"("error in (no error)"=w9050, "State Machine.lvclass"=w9048, "Device in"=w9049) -> ("error out"=w9054:errorcluster, "Device out"=w9055:refnum<class "Channel.lvclass">)  [unwired: 7 in]
            n3824 = call-dynamic "Write Channel.vi"("error in (no error)"=w9054, "Channel.lvclass"=w9055, "Acquisition in"=w9053) -> ("error out"=w9052:errorcluster, "Acquisition out"=w9051:refnum<class "Acquisition.lvclass">)  [unwired: 7 in]
            n3825 = call-dynamic "Write AcquisitionA.vi"("error in (no error)"=w9052, "Acquisition.lvclass"=w9051, "S4ACS_GUI in"=w9039) -> ("error out"=w9024:errorcluster, "S4ACS_GUI out"=w9023:refnum<class "S4GUI.lvclass">)  [unwired: 7 in]
            n3826 = call "Read AcquisitionB.vi"("error in (no error)"=w9024, "S4ACS_GUI in"=w9023) -> ("error out"=w9017:errorcluster, "Acquisition.lvclass"=w9021:refnum<class "Acquisition.lvclass">, "S4ACS_GUI out"=w9022:refnum<class "S4GUI.lvclass">)  [unwired: 7 in]
            n3827 = call-dynamic "Read Channel.vi"("error in (no error)"=w9017, "Acquisition in"=w9021) -> ("error out"=w9032:errorcluster, "Channel.lvclass"=w9033:refnum<class "Channel.lvclass">, "Acquisition out"=w9019:refnum<class "Acquisition.lvclass">)  [unwired: 7 in]
            n3828 = call-dynamic "Read State Machine.vi"("error in (no error)"=w9032, "Device in"=w9033) -> ("error out"=w9030:errorcluster, "State Machine.lvclass"=w9031:refnum<class "State Machine.lvclass">, "Device out"=w9028:refnum<class "Channel.lvclass">)  [unwired: 7 in]
            n3829 = call "Next State.vi"("error in (no error)"=w9030, "New_State"=u32 80, "State Machine in"=w9031) -> ("error out"=w9027:errorcluster, "State Machine out"=w9029:refnum<class "State Machine.lvclass">)  [unwired: 7 in]
            n3830 = call-dynamic "Write State Machine.vi"("error in (no error)"=w9027, "State Machine.lvclass"=w9029, "Device in"=w9028) -> ("error out"=w9026:errorcluster, "Device out"=w9025:refnum<class "Channel.lvclass">)  [unwired: 7 in]
            n3831 = call-dynamic "Write Channel.vi"("error in (no error)"=w9026, "Channel.lvclass"=w9025, "Acquisition in"=w9019) -> ("error out"=w9018:errorcluster, "Acquisition out"=w9020:refnum<class "Acquisition.lvclass">)  [unwired: 7 in]
            n3832 = call "Write AcquisitionB.vi"("error in (no error)"=w9018, "Acquisition.lvclass"=w9020, "S4ACS_GUI in"=w9022) -> ("error out"=w8984:errorcluster, "S4ACS_GUI out"=w8983:refnum<class "S4GUI.lvclass">)  [unwired: 7 in]
            n3833 = call-dynamic "Read AcquisitionC.vi"("error in (no error)"=w8984, "S4ACS_GUI in"=w8983) -> ("error out"=w9001:errorcluster, "Acquisition.lvclass"=w9005:refnum<class "Acquisition.lvclass">, "S4ACS_GUI out"=w9006:refnum<class "S4GUI.lvclass">)  [unwired: 7 in]
            n3834 = call-dynamic "Read Channel.vi"("error in (no error)"=w9001, "Acquisition in"=w9005) -> ("error out"=w9014:errorcluster, "Channel.lvclass"=w9015:refnum<class "Channel.lvclass">, "Acquisition out"=w9003:refnum<class "Acquisition.lvclass">)  [unwired: 7 in]
            n3835 = call-dynamic "Read State Machine.vi"("error in (no error)"=w9014, "Device in"=w9015) -> ("error out"=w9012:errorcluster, "State Machine.lvclass"=w9013:refnum<class "State Machine.lvclass">, "Device out"=w9010:refnum<class "Channel.lvclass">)  [unwired: 7 in]
            n3836 = call "Next State.vi"("error in (no error)"=w9012, "New_State"=u32 80, "State Machine in"=w9013) -> ("error out"=w9009:errorcluster, "State Machine out"=w9011:refnum<class "State Machine.lvclass">)  [unwired: 7 in]
            n3837 = call-dynamic "Write State Machine.vi"("error in (no error)"=w9009, "State Machine.lvclass"=w9011, "Device in"=w9010) -> ("error out"=w9008:errorcluster, "Device out"=w9007:refnum<class "Channel.lvclass">)  [unwired: 7 in]
            n3838 = call-dynamic "Write Channel.vi"("error in (no error)"=w9008, "Channel.lvclass"=w9007, "Acquisition in"=w9003) -> ("error out"=w9002:errorcluster, "Acquisition out"=w9004:refnum<class "Acquisition.lvclass">)  [unwired: 7 in]
            n3839 = call-dynamic "Write AcquisitionC.vi"("error in (no error)"=w9002, "Acquisition.lvclass"=w9004, "S4ACS_GUI in"=w9006) -> ("error out"=w8982:errorcluster, "S4ACS_GUI out"=w8981:refnum<class "S4GUI.lvclass">)  [unwired: 7 in]
            n3840 = call-dynamic "Read AcquisitionD.vi"("error in (no error)"=w8982, "S4ACS_GUI in"=w8981) -> ("error out"=w8985:errorcluster, "Acquisition.lvclass"=w8989:refnum<class "Acquisition.lvclass">, "S4ACS_GUI out"=w8990:refnum<class "S4GUI.lvclass">)  [unwired: 7 in]
            n3841 = call-dynamic "Read Channel.vi"("error in (no error)"=w8985, "Acquisition in"=w8989) -> ("error out"=w8998:errorcluster, "Channel.lvclass"=w8999:refnum<class "Channel.lvclass">, "Acquisition out"=w8987:refnum<class "Acquisition.lvclass">)  [unwired: 7 in]
            n3842 = call-dynamic "Read State Machine.vi"("error in (no error)"=w8998, "Device in"=w8999) -> ("error out"=w8996:errorcluster, "State Machine.lvclass"=w8997:refnum<class "State Machine.lvclass">, "Device out"=w8994:refnum<class "Channel.lvclass">)  [unwired: 7 in]
            n3843 = call "Next State.vi"("error in (no error)"=w8996, "New_State"=u32 80, "State Machine in"=w8997) -> ("error out"=w8993:errorcluster, "State Machine out"=w8995:refnum<class "State Machine.lvclass">)  [unwired: 7 in]
            n3844 = call-dynamic "Write State Machine.vi"("error in (no error)"=w8993, "State Machine.lvclass"=w8995, "Device in"=w8994) -> ("error out"=w8992:errorcluster, "Device out"=w8991:refnum<class "Channel.lvclass">)  [unwired: 7 in]
            n3845 = call-dynamic "Write Channel.vi"("error in (no error)"=w8992, "Channel.lvclass"=w8991, "Acquisition in"=w8987) -> ("error out"=w8986:errorcluster, "Acquisition out"=w8988:refnum<class "Acquisition.lvclass">)  [unwired: 7 in]
            n3846 = call-dynamic "Write AcquisitionD.vi"("error in (no error)"=w8986, "Acquisition.lvclass"=w8988, "S4ACS_GUI in"=w8990) -> ("error out"=w8979:errorcluster, "S4ACS_GUI out"=w8980:refnum<class "S4GUI.lvclass">)  [unwired: 7 in]
            n3847 = disable-structure shown="Enabled" {
              disable-tunnel: w8980 -> [w9060 w9062]
              disable-tunnel: w8979 -> [w9059 w9061]
              disable-tunnel: [w9057 w9062] -> w9036
              disable-tunnel: [w9056 w9061] -> w9035
              frame Disabled {
                n3848 = call-dynamic "Write aborted.vi"("error in (no error)"=w9059, "aborted"=TRUE ("stopped"), "S4ACS_GUI in"=w9060) -> ("error out"=w9056:errorcluster, "S4ACS_GUI out"=w9057:refnum<class "S4GUI.lvclass">)  [unwired: 7 in]
              }
              frame Enabled {
              }
            }
            n3849 = call-dynamic "Write Obs_state.vi"("error in (no error)"=w9035, "Obs_state"=u32 0, "S4ACS_GUI in"=w9036) -> ("error out"=w8953:errorcluster, "S4ACS_GUI out"=w8954:refnum<class "S4GUI.lvclass">)  [unwired: 7 in]
            n3850 = call "Read Instrument.lvclass.vi"("error in (no error)"=w8953, "S4ACS_GUI in"=w8954) -> ("error out"=w8973:errorcluster, "Instrument.lvclass"=w8975:refnum<class "Instrument.lvclass">, "S4ACS_GUI out"=w8974:refnum<class "S4GUI.lvclass">)  [unwired: 7 in]
            n3851 = call "Read WPROT.vi"("error in (no error)"=w8973, "Instrument in"=w8975) -> ("error out"=w8968:errorcluster, "Opt_Selector.lvclass"=w8971:refnum<class "Opt_Selector.lvclass">, "Instrument out"=w8976:refnum<class "Instrument.lvclass">)  [unwired: 7 in]
            n3852 = call-dynamic "Read sequencia_ant.vi"("error in (no error)"=w8968, "Opt_Selector in"=w8971) -> ("error out"=w8967:errorcluster, "sequencia_ant"=w8969:u16, "Opt_Selector out"=w8970:refnum<class "Opt_Selector.lvclass">)  [unwired: 7 in]
